vi "Raycaster_SetupDDA.vi"(10 "Camera X":fxp<+/-,32,16> format="%#_21g", 11 "Location Info (Axis)":T2) -> (3 "Wall Column (Axis)":T1)   [LabVIEW 2020]
uses:
  Controls/Player_LocationInfoAxis.ctl
  Controls/Raycaster_WallColumnAxis.ctl
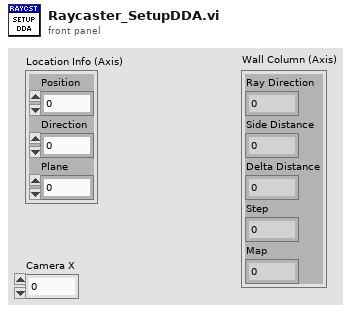
[diagram p1: front panel]
types:
  T1 = typedef "Raycaster_WallColumnAxis.ctl" = cluster{"Ray Direction":fxp<+/-,32,16>, "Side Distance":fxp<+/-,32,16>, "Delta Distance":fxp<+/-,32,16>, "Step":i16, "Map":i16}
  T2 = typedef "Player_LocationInfoAxis.ctl" = cluster{"Position":fxp<+/-,32,16>, "Direction":fxp<+/-,32,16>, "Plane":fxp<+/-,32,16>}
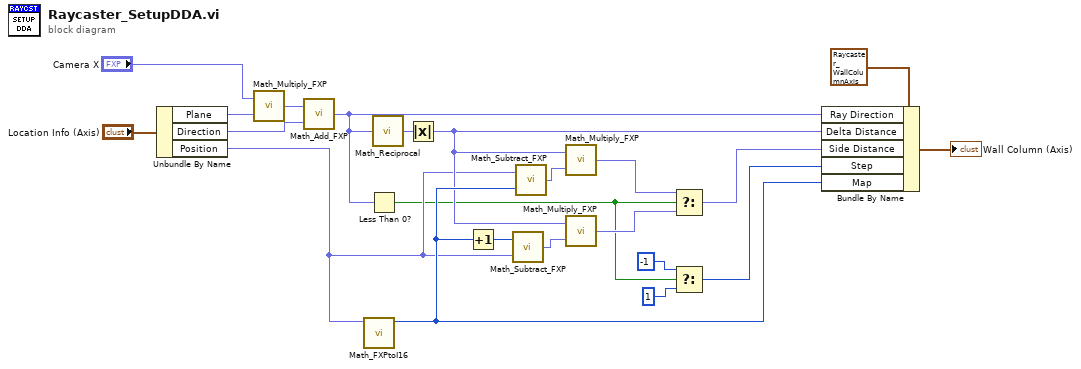
[diagram p0: block diagram]
diagram:
  n1 = Unbundle By Name("Location Info (Axis)") -> ("Plane"=w19:fxp<+/-,32,16>, "Direction"=w16:fxp<+/-,32,16>, "Position"=w9:fxp<+/-,32,16>)
  n2 = call "Math_Multiply_FXP.vi"("y"=w19, "x"="Camera X") -> ("x*y"=w17:fxp<+/-,32,16>)
  n3 = call "Math_Add_FXP.vi"("y"=w16, "x"=w17) -> ("x*y"=w14:fxp<+/-,32,16>)
  n4 = call "Math_FXPtoI16.vi"("FXP"=w9) -> ("I16"=w11:i16)  [unwired: 10 in]
  n5 = Less Than 0?(x=w14) -> (x < 0?=w5:bool)
  n6 = call "Math_Reciprocal.vi"("x"=w14) -> ("1/x"=w15:fxp<+/-,32,16>)
  n7 = Absolute Value(x=w15) -> (abs(x)=w10:fxp<+,32,16>)
  n8 = Increment(x=w11) -> (x+1=w12:i16)
  n9 = call "Math_Subtract_FXP.vi"("y"=w9, "x"=w12) -> ("x*y"=w13:fxp<+/-,32,16>)
  n10 = call "Math_Subtract_FXP.vi"("y"=w11, "x"=w9) -> ("x*y"=w8:fxp<+/-,32,16>)
  n11 = call "Math_Multiply_FXP.vi"("y"=w8, "x"=w10) -> ("x*y"=w7:fxp<+/-,32,16>)
  n12 = call "Math_Multiply_FXP.vi"("y"=w13, "x"=w10) -> ("x*y"=w6:fxp<+/-,32,16>)
  n13 = Select(t=w7, s=w5, f=w6) -> (s? t:f=w1:fxp<+/-,32,16>)
  n14 = Select(t=i16 -1 ("Step"), s=w5, f=i16 1 ("Step")) -> (s? t:f=w2:i16)
  n15 = Bundle By Name(cluster=T1 {"Ray Direction"=0.0, "Side Distance"=0.0, "Delta Distance"=0.0, "Step"=0, "Map"=0} ("Wall Column (Axis)"), "Ray Direction"=w14, "Delta Distance"=w10, "Side Distance"=w1, "Step"=w2, "Map"=w11) -> (→"Wall Column (Axis)":T1)
